vi "TM_datasocket3.vi"() -> ()   [LabVIEW 2018]
panel:
  out "水平进度条":dbl(slide) scale=0.0..100.0
  out "数据":cdb[](array[numeric])
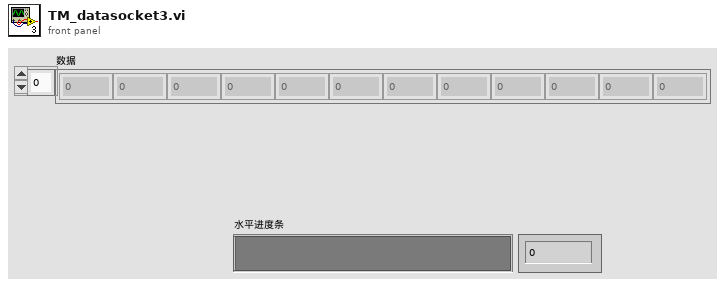
[diagram p1: front panel]
types:
  T1 = enum16{"Read", "Write", "ReadWrite", "BufferedRead", "BufferedReadWrite"}
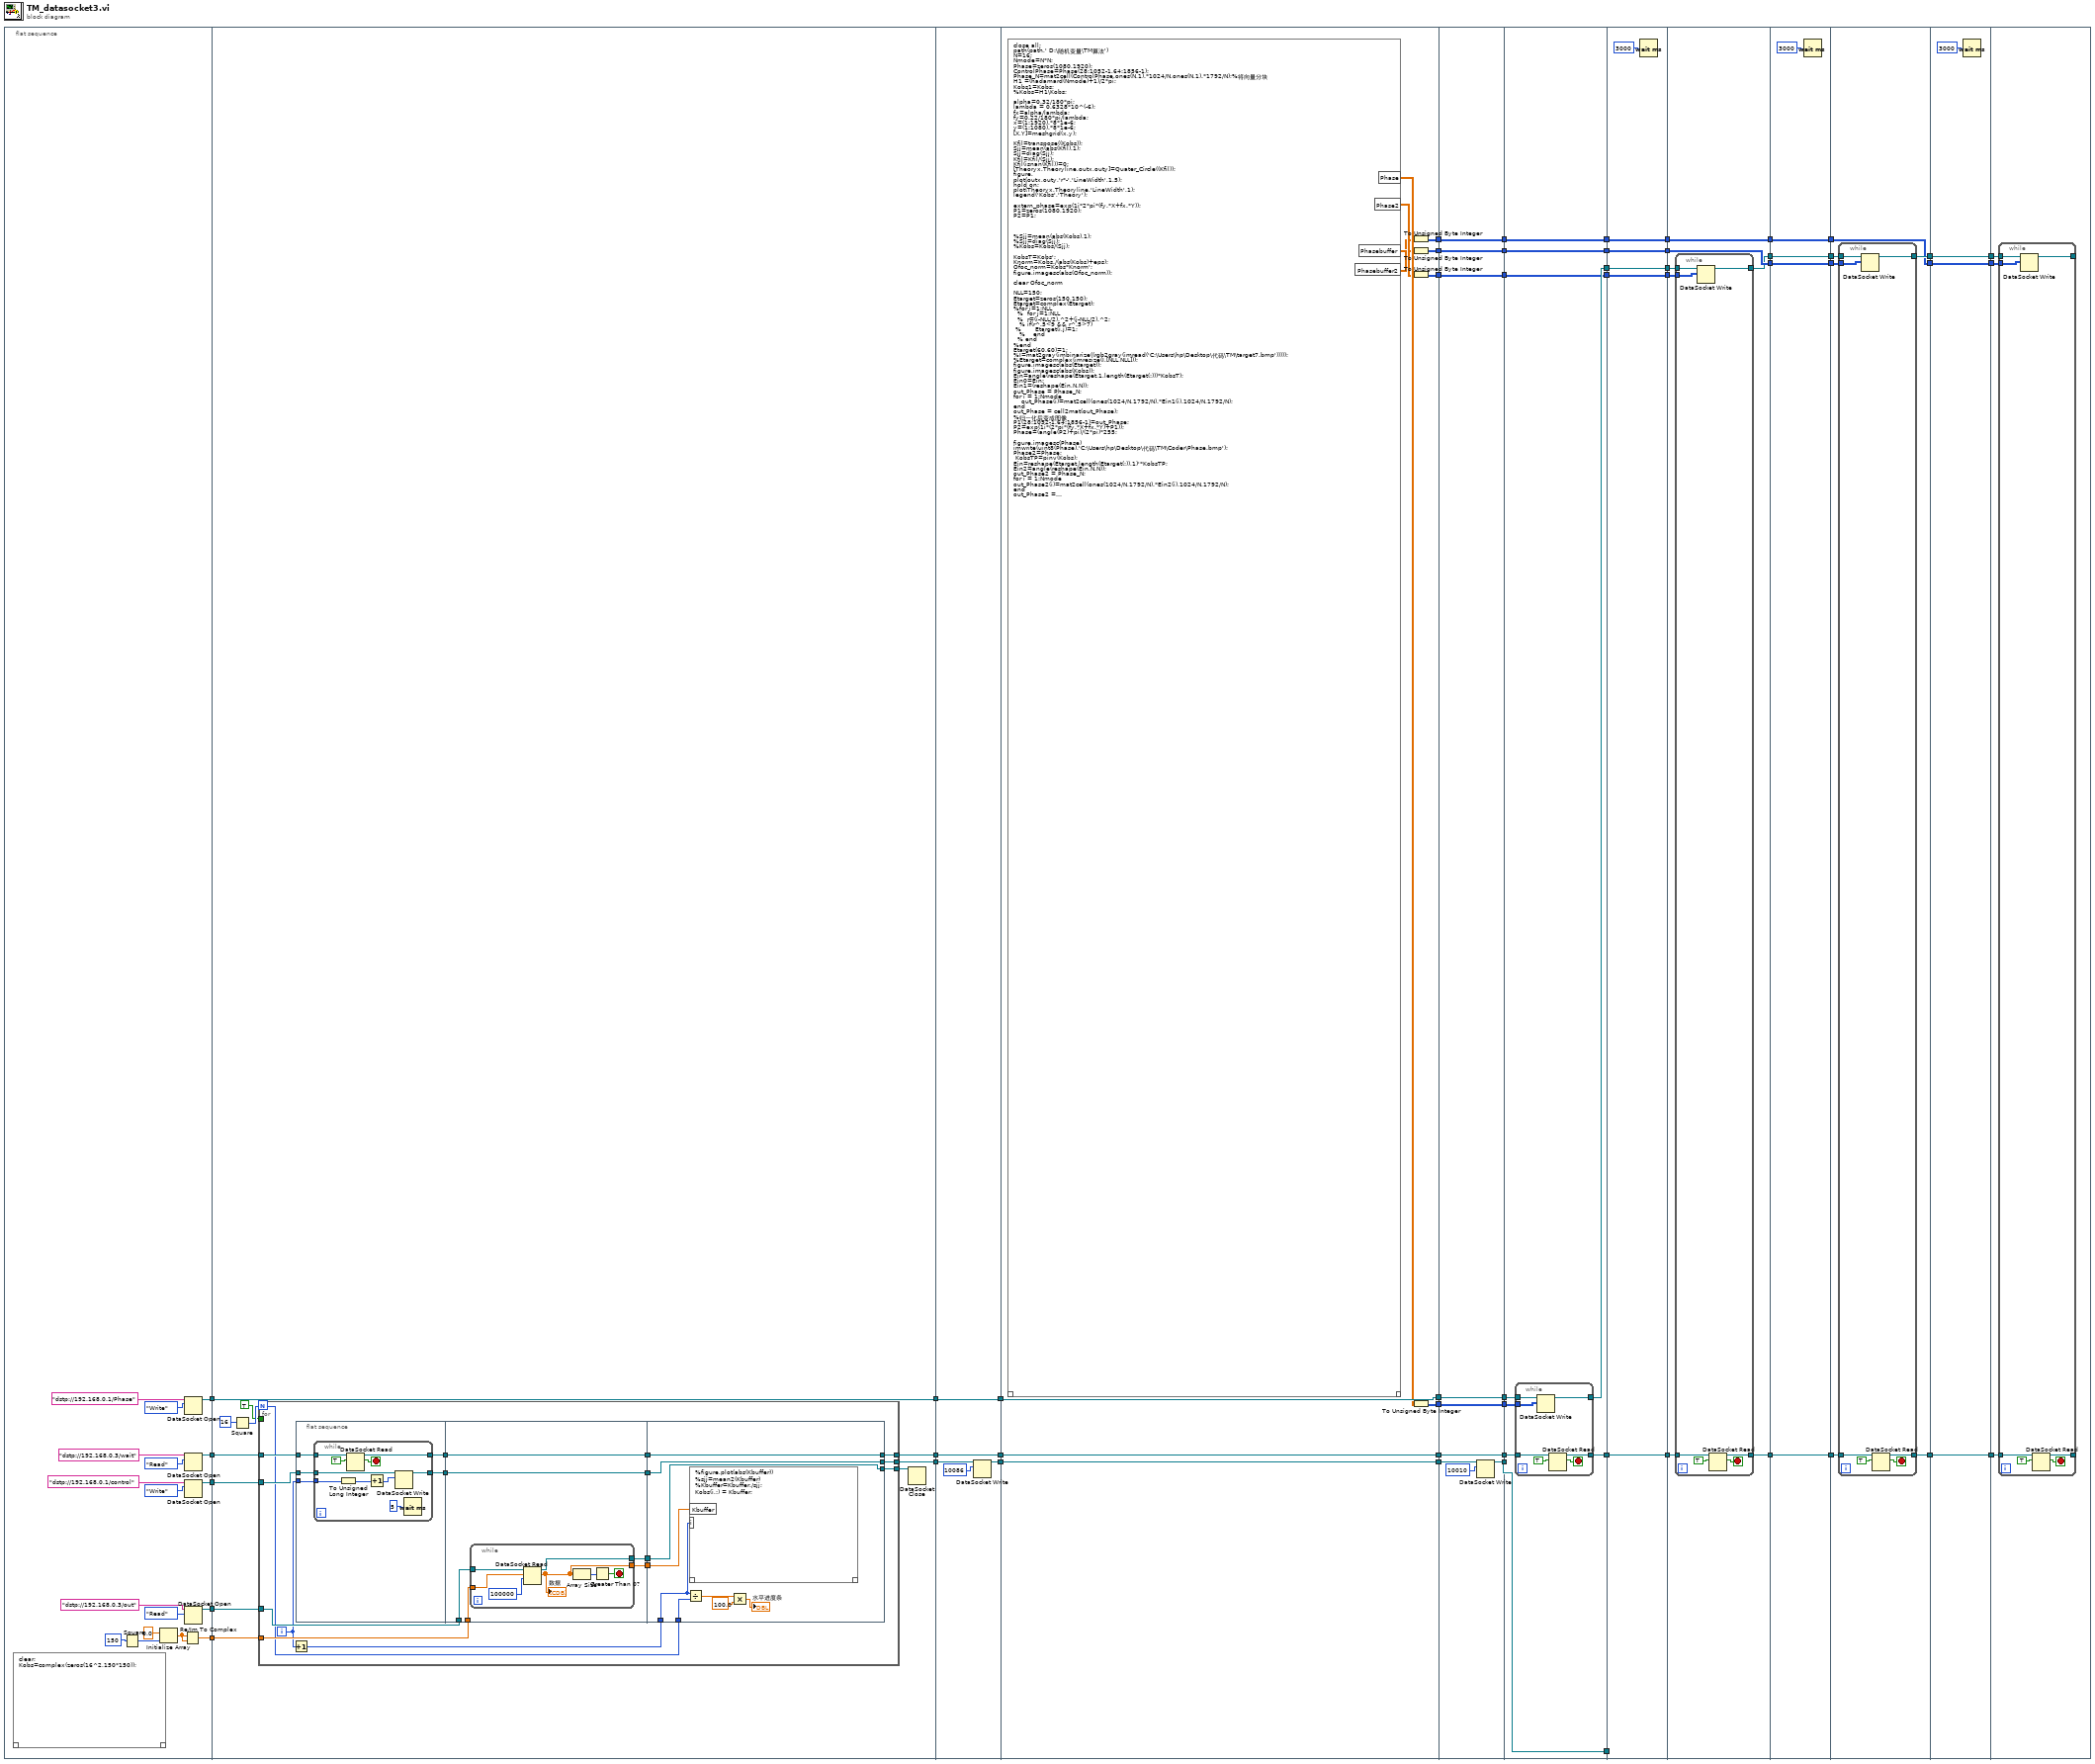
[diagram p0: block diagram]
diagram:
  n1 = flat-sequence {
    tunnel: [w63] -> w50
    tunnel: [w62] -> w49
    tunnel: [w56] -> w48
    tunnel: [w54] -> w47
    tunnel: [w51] -> w46
    tunnel: w50 -> [w76]
    tunnel: w49 -> [w75]
    tunnel: w48 -> [w71]
    tunnel: w47 -> [w74]
    tunnel: [w70] -> w45
    tunnel: w46 -> [w70]
    tunnel: [w69] -> w43
    tunnel: [w68] -> w35
    tunnel: w45 -> [w136]
    tunnel: [w136] -> w44
    tunnel: w43 -> [w135]
    tunnel: [w133] -> w37
    tunnel: [w132] -> w36
    tunnel: w35 -> [w132]
    tunnel: w44 -> [w147]
    tunnel: [w147] -> w42
    tunnel: [w145] -> w40
    tunnel: [w144] -> w38
    tunnel: w37 -> [w144]
    tunnel: w36 -> [w143]
    tunnel: [w143] -> w33
    tunnel: [w141] -> w26
    tunnel: [w139] -> w19
    tunnel: [w137] -> w1
    tunnel: w42 -> [w156]
    tunnel: [w156] -> w41
    tunnel: w40 -> [w155]
    tunnel: [w155] -> w39
    tunnel: w38 -> [w153]
    tunnel: [w152] -> w34
    tunnel: w33 -> [w152]
    tunnel: [w151] -> w31
    tunnel: w26 -> [w150]
    tunnel: [w150] -> w25
    tunnel: [w149] -> w20
    tunnel: w19 -> [w149]
    tunnel: [w148] -> w2
    tunnel: w1 -> [w148]
    tunnel: w41 -> [w164]
    tunnel: w39 -> [w165]
    tunnel: w34 -> [w163]
    tunnel: [w162] -> w32
    tunnel: w31 -> [w162]
    tunnel: [w161] -> w30
    tunnel: [w160] -> w27
    tunnel: w25 -> [w159]
    tunnel: [w159] -> w24
    tunnel: [w158] -> w21
    tunnel: w20 -> [w158]
    tunnel: [w157] -> w3
    tunnel: w2 -> [w157]
    tunnel: w32 -> [_]
    tunnel: w30 -> [w177]
    tunnel: [w177] -> w29
    tunnel: [w176] -> w28
    tunnel: w27 -> [w176]
    tunnel: w24 -> [w175]
    tunnel: [w175] -> w23
    tunnel: [w174] -> w22
    tunnel: w21 -> [w174]
    tunnel: [w173] -> w4
    tunnel: w3 -> [w173]
    tunnel: w29 -> [w185]
    tunnel: w28 -> [w184]
    tunnel: w23 -> [w183]
    tunnel: w22 -> [w182]
    tunnel: [w182] -> w18
    tunnel: [w181] -> w16
    tunnel: [w180] -> w14
    tunnel: [w179] -> w5
    tunnel: w4 -> [w179]
    tunnel: w18 -> [w197]
    tunnel: [w197] -> w17
    tunnel: w16 -> [w195]
    tunnel: [w195] -> w15
    tunnel: w14 -> [w194]
    tunnel: [w194] -> w13
    tunnel: [w193] -> w6
    tunnel: w5 -> [w193]
    tunnel: w17 -> [w203]
    tunnel: w15 -> [w202]
    tunnel: w13 -> [w201]
    tunnel: [w200] -> w12
    tunnel: [w199] -> w10
    tunnel: [w198] -> w7
    tunnel: w6 -> [w198]
    tunnel: w12 -> [w213]
    tunnel: [w213] -> w11
    tunnel: w10 -> [w212]
    tunnel: [w212] -> w9
    tunnel: [w211] -> w8
    tunnel: w7 -> [w211]
    tunnel: w11 -> [w217]
    tunnel: w9 -> [w216]
    tunnel: w8 -> [w215]
    frame #0 {
      n2 = script code="clear;\nKobs=complex(zeros(16^2,150*150));"() -> ()  [unwired: 1 in, 1 out]
      n3 = Square(x=150 ("维数大小")) -> (x^2=w59:i32)
      n4 = Initialize Array(0.0 ("元素"), w59) -> (w55:dbl[])
      n5 = Re/Im To Complex(1:w55, 2:w55) -> (0:w54:cdb[])
      n6 = DataSocket Open(10:T1."Write" ("模式"), 11:"dstp://192.168.0.1/Phase" ("URL")) -> (3:w51:refnum<k13>)  [unwired: 2 in, 1 out]
      n7 = DataSocket Open(10:T1."Read" ("模式"), 11:"dstp://192.168.0.3/wait" ("URL")) -> (3:w56:refnum<k13>)  [unwired: 2 in, 1 out]
      n8 = DataSocket Open(10:T1."Write" ("模式"), 11:"dstp://192.168.0.1/control" ("URL")) -> (3:w63:refnum<k13>)  [unwired: 2 in, 1 out]
      n9 = DataSocket Open(10:T1."Read" ("模式"), 11:"dstp://192.168.0.3/out" ("URL")) -> (3:w62:refnum<k13>)  [unwired: 2 in, 1 out]
    }
    frame #1 {
      n10 = Square(x=16) -> (x^2=w77:i32)
      n11 = for {
        N: w77 -> [w79]
        tunnel: w76 -> [w81]
        tunnel: [w94] -> w69
        tunnel: w75 -> [w93]
        tunnel: w74 -> [w92]
        tunnel: [w91] -> w73
        tunnel: TRUE -> [_]
        tunnel: w71 -> [w86]
        tunnel: [w83] -> w68
        i -> [w82]
        n12 = Increment(x=w82) -> (x+1=w80:i32)
        n13 = flat-sequence {
          tunnel: [w95] -> w87
          tunnel: [w98] -> w84
          tunnel: w82 -> [w97]
          tunnel: w81 -> [w96]
          tunnel: w86 -> [w99]
          tunnel: w87 -> [w115]
          tunnel: w93 -> [w114]
          tunnel: w92 -> [w113]
          tunnel: [w115] -> w90
          tunnel: [w112] -> w89
          tunnel: [w111] -> w88
          tunnel: [w110] -> w85
          tunnel: w84 -> [w110]
          tunnel: [w130] -> w91
          tunnel: [w131] -> w94
          tunnel: w90 -> [w131]
          tunnel: w89 -> [w130]
          tunnel: w88 -> [w129]
          tunnel: w80 -> [w127]
          tunnel: [w128] -> w83
          tunnel: w85 -> [w128]
          tunnel: w79 -> [w126]
          frame #0 {
            n14 = while {
              tunnel: w99 -> [w109]
              tunnel: [w106] -> w98
              tunnel: w97 -> [w103]
              tunnel: w96 -> [w102]
              tunnel: [w101] -> w95
              stop <- w107 stop-if-true
              n15 = To Unsigned Long Integer(number=w103) -> (unsigned 32bit integer=w105:u32)
              n16 = DataSocket Read(10:TRUE, 11:w109) -> (2:w107:bool, 3:w106:refnum<k13>)  [unwired: 3 in, 5 out]
              n17 = Increment(x=w105) -> (x+1=w104:u32)
              n18 = DataSocket Write(10:w104, 11:w102) -> (3:w101:refnum<k13>)  [unwired: 2 in, 2 out]
              n19 = Wait (ms)(milliseconds to wait=u32 5 ("等待时间（毫秒）")) -> ()  [unwired: 1 out]
            }
          }
          frame #1 {
            n20 = while {
              tunnel: w114 -> [w122]
              tunnel: [w120] -> w112
              tunnel: w113 -> [w121]
              tunnel: [w118] -> w111
              stop <- w116 stop-if-true
              n21 = DataSocket Read(9:100000 ("毫秒超时(10000)"), 10:w121, 11:w122) -> (2:w118:cdb[], 3:w120:refnum<k13>)  [unwired: 2 in, 5 out]
              "数据" <- w118
              n22 = Array Size(array=w118) -> (size(s)=w117:i32)
              n23 = Greater Than 0?(x=w117) -> (x > 0?=w116:bool)
            }
          }
          frame #2 {
            n24 = Divide(x=w127, y=w126) -> (x/y=w125:dbl)
            n25 = script code="%figure,plot(abs(Kbuffer))\n%sjj=mean2(Kbuffer)\n%Kbuffer=Kbuffer./sjj;\nKobs(i,:) = Kbuffer;"("Kbuffer"=w129, "i"=w127) -> ()  [unwired: 1 in, 1 out]
            n26 = Multiply(x=w125, y=100.0) -> (x*y=→"水平进度条":dbl)
          }
        }
      }
      n27 = DataSocket Close(11:w73) -> ()  [unwired: 2 in, 2 out]
    }
    frame #2 {
      n28 = DataSocket Write(10:10086, 11:w135) -> (3:w133:refnum<k13>)  [unwired: 2 in, 2 out]
    }
    frame #3 {
      n29 = script code="close all;\npath(path,' D:\\随机变量\\TM算法')\nN=16;\nNmode=N*N;\nPhase=zeros(1080,1920);\nControlPhase=Phase(28:1052-1,64:1856-1);\nPhase_N=mat2cell(ControlPhase,ones(N,1).*1024/N,ones(N,1).*1792/N);%将向量分块\nH1 =(hadamard(Nmode)+1)/2*pi; \nKobs1=Kobs;\n%Kobs=H1\\Kobs;\n\nalpha=0.32/180*pi;\nlambda = 0.6328*10^(-6);\nfx=alpha/lambda;\nfy=0.22/180*pi/lambda;\nx=(1:1920).*8*1e-6;\ny=(1:1080).*8*1e-6;\n[X,Y]=meshgrid(x,y);\n\nKfil=transpose((Kobs));\nSjj=mean(abs(Kfil),1); \nSjj=diag(Sjj);\nKfil=Kfil/(Sjj);\nKfil(isnan(Kfil))=0;\n[Theoryx,Theoryline,outx,outy]=Quater_Circle((Kfil));\nfigure,\nplot(outx,outy,'r*-','LineWidth',1.5);\nhold on;\nplot(Theoryx,Theoryline,'LineWidth',1);\nlegend('Kobs','Theory');\n\nextern_phase=exp(1i*2*pi*(fy.*X+fx.*Y));\nP1=zeros(1080,1920);\nP2=P1;\n\n\n\n%Sjj=mean(abs(Kobs),1);\n%Sjj=diag(Sjj);\n%Kobs=Kobs/(Sjj);\n\nKobsT=Kobs';\nKnorm=Kobs./(abs(Kobs)+eps);\nOfoc_norm=Kobs*Knorm';\nfigure,imagesc(abs(Ofoc_norm));\n\nclear Ofoc_norm\n\nNLL=150;\nEtarget=zeros(150,150);\nEtarget=complex(Etarget);\n%for i=1:NLL\n  %  for j=1:NLL\n  %  r=(i-NLL/2).^2+(j-NLL/2).^2;\n   % if(r^.5<9 && r^.5>7)\n %       Etarget(i,j)=1;\n   %    end\n  % end\n%end\nEtarget(60,60)=1;\n%I=mat2gray(imbinarize((rgb2gray(imread('C:\\Users\\hp\\Desktop\\代码\\TM\\target7.bmp')))));\n%Etarget=complex(imresize(I,[NLL,NLL]));\nfigure,imagesc(abs(Etarget));\nfigure,imagesc(abs(Kobs));\nEin=angle(reshape(Etarget,1,length(Etarget(:)))*KobsT);\nEin0=Ein;\nEin1=(reshape(Ein,N,N));\nout_Phase = Phase_N;\nfor i = 1:Nmode\n    out_Phase(i)=mat2cell(ones(1024/N,1792/N).*Ein1(i),1024/N,1792/N);\nend\nout_Phase = cell2mat(out_Phase);\n%归一化后变成图像\nP1(28:1052-1,64:1856-1)=out_Phase;\nP2=exp(1i*(2*pi*(fy.*X+fx.*Y)+P1));\nPhase=(angle(P2)+pi)/(2*pi)*255;\n\nfigure,imagesc(Phase)\nimwrite(uint8(Phase),'C:\\Users\\hp\\Desktop\\代码\\TM\\Coder\\Phase.bmp');\nPhase2=Phase;\n KobsTP=pinv(Kobs);\nEin=reshape(Etarget,length(Etarget(:)),1)'*KobsTP;\nEin2=angle(reshape(Ein,N,N));\nout_Phase2 = Phase_N;\nfor i = 1:Nmode\nout_Phase2(i)=mat2cell(ones(1024/N,1792/N).*Ein2(i),1024/N,1792/N);\nend\nout_Phase2 = cell2mat(out_Phase2);\nP1(28:1052-1,64:1856-1)=out_Phase2;\nP2=exp(1i*(2*pi*(fy.*X+fx.*Y)+P1));\nPhase2=(angle(P2)+pi)/(2*pi)*255;\n\nfigure,imagesc(Phase2)\nimwrite(uint8(Phase2),'C:\\Users\\hp\\Desktop\\代码\\TM\\Coder\\Phase2.bmp');\n\ninter=2000;\nU0=ones(size(Phase2)).*exp(1i*Phase2);\nPhasebuffer=Phase2;\nUinverse_phase=angle(Ein)+pi;\nEtarget1=reshape(Etarget,length(Etarget(:)),1);\nfor k=1:inter\n \n    Uout=(ones(length(Uinverse_phase),1)'*255.*exp(1i*Uinverse_phase))*Kobs;\n    Uinverse_in=exp(1i*angle(Uout)).*abs(Etarget1)';\n    Uinverse_out=Uinverse_in*KobsTP;\n    Uinverse_phase=angle(Uinverse_out);\n\nend\nUout=reshape(Uout,NLL,NLL);\nfigure,imagesc(abs(Uout));\nout_Phasebuffer = Phase_N;\n    for i = 1:Nmode\n      out_Phasebuffer(i)=mat2cell(ones(1024/N,1792/N).*Uinverse_phase(i),1024/N,1792/N);\n    end\nout_Phasebuffer = cell2mat(out_Phasebuffer);\nP1(28:1052-1,64:1856-1)=out_Phasebuffer;\nP2=exp(1i*(2*pi*(fy.*X+fx.*Y)+P1));\nPhasebuffer=(angle(P2)+pi)/(2*pi)*255;\n\n\nfigure,imagesc(Phasebuffer)\nimwrite(uint8(Phasebuffer),'C:\\Users\\hp\\Desktop\\代码\\TM\\Coder\\Phasebuffer2000.bmp');\n\n\nAout=Y_G_Algorithm(Kobs,Etarget1,angle(Ein)+pi,inter);\nout_Phasebuffer2= Phase_N;\nfor i = 1:Nmode\n      out_Phasebuffer2(i)=mat2cell(ones(1024/N,1792/N).*Aout(i),1024/N,1792/N);\n end\nout_Phasebuffer2 = cell2mat(out_Phasebuffer2);\nP1(28:1052-1,64:1856-1)=out_Phasebuffer2;\nP2=exp(1i*(2*pi*(fy.*X+fx.*Y)+P1));\nPhasebuffer2=(angle(P2)+pi)/(2*pi)*255;\n\nimwrite(uint8(Phasebuffer2),'C:\\Users\\hp\\Desktop\\代码\\TM\\Coder\\Phasebuffer22000.bmp');"() -> ("Phase"=w146:dbl[][], "Phase2"=w142:dbl[][], "Phasebuffer"=w140:dbl[][], "Phasebuffer2"=w138:dbl[][])  [unwired: 1 in, 1 out]
      n30 = To Unsigned Byte Integer(number=w138) -> (unsigned 8bit integer=w137:u8[][])
      n31 = To Unsigned Byte Integer(number=w140) -> (unsigned 8bit integer=w139:u8[][])
      n32 = To Unsigned Byte Integer(number=w142) -> (unsigned 8bit integer=w141:u8[][])
      n33 = To Unsigned Byte Integer(number=w146) -> (unsigned 8bit integer=w145:u8[][])
    }
    frame #4 {
      n34 = DataSocket Write(10:10010, 11:w153) -> (3:w151:refnum<k13>)  [unwired: 2 in, 2 out]
    }
    frame #5 {
      n35 = while {
        tunnel: w165 -> [w172]
        tunnel: w163 -> [w169]
        tunnel: [w166] -> w160
        tunnel: w164 -> [w170]
        tunnel: [w171] -> w161
        stop <- w167 stop-if-true
        n36 = DataSocket Write(10:w172, 11:w170) -> (3:w171:refnum<k13>)  [unwired: 2 in, 2 out]
        n37 = DataSocket Read(10:TRUE, 11:w169) -> (2:w167:bool, 3:w166:refnum<k13>)  [unwired: 3 in, 5 out]
      }
    }
    frame #6 {
      n38 = Wait (ms)(milliseconds to wait=u32 3000 ("等待时间（毫秒）")) -> ()  [unwired: 1 out]
    }
    frame #7 {
      n39 = while {
        tunnel: w183 -> [w192]
        tunnel: w184 -> [w189]
        tunnel: [w186] -> w180
        tunnel: w185 -> [w190]
        tunnel: [w191] -> w181
        stop <- w187 stop-if-true
        n40 = DataSocket Write(10:w192, 11:w190) -> (3:w191:refnum<k13>)  [unwired: 2 in, 2 out]
        n41 = DataSocket Read(10:TRUE, 11:w189) -> (2:w187:bool, 3:w186:refnum<k13>)  [unwired: 3 in, 5 out]
      }
    }
    frame #8 {
      n42 = Wait (ms)(milliseconds to wait=u32 3000 ("等待时间（毫秒）")) -> ()  [unwired: 1 out]
    }
    frame #9 {
      n43 = while {
        tunnel: w203 -> [w210]
        tunnel: w201 -> [w207]
        tunnel: [w204] -> w199
        tunnel: w202 -> [w208]
        tunnel: [w209] -> w200
        stop <- w205 stop-if-true
        n44 = DataSocket Write(10:w210, 11:w208) -> (3:w209:refnum<k13>)  [unwired: 2 in, 2 out]
        n45 = DataSocket Read(10:TRUE, 11:w207) -> (2:w205:bool, 3:w204:refnum<k13>)  [unwired: 3 in, 5 out]
      }
    }
    frame #10 {
      n46 = Wait (ms)(milliseconds to wait=u32 3000 ("等待时间（毫秒）")) -> ()  [unwired: 1 out]
    }
    frame #11 {
      n47 = while {
        tunnel: w215 -> [w224]
        tunnel: w216 -> [w221]
        tunnel: [w218] -> _
        tunnel: w217 -> [w222]
        tunnel: [w223] -> _
        stop <- w219 stop-if-true
        n48 = DataSocket Write(10:w224, 11:w222) -> (3:w223:refnum<k13>)  [unwired: 2 in, 2 out]
        n49 = DataSocket Read(10:TRUE, 11:w221) -> (2:w219:bool, 3:w218:refnum<k13>)  [unwired: 3 in, 5 out]
      }
    }
  }
